vi "ComplexClusterControls.vi"() -> ()   [LabVIEW 2016, in "test_ValueSignal.lvlib"]
uses:
  test_ValueSignal.lvlib
  Helper/HelperVI1.vi
  main/apis/Stimulus/ValueSignalByName.vi
  main/apis/Assert/AssertControlValueByName.vi
  <vilib>/addons/_JKI Toolkits/Caraya/classes/Assert/Assert Equal Value_Variant.vi
  <vilib>/addons/_JKI Toolkits/Caraya/classes/Assert/Assert.lvclass
  <vilib>/addons/_JKI Toolkits/Caraya/classes/Test/Test.lvclass
panel:
  out "error out":errorcluster
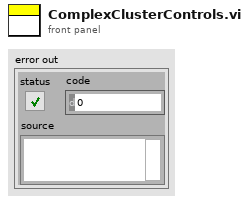
[diagram p1: front panel]
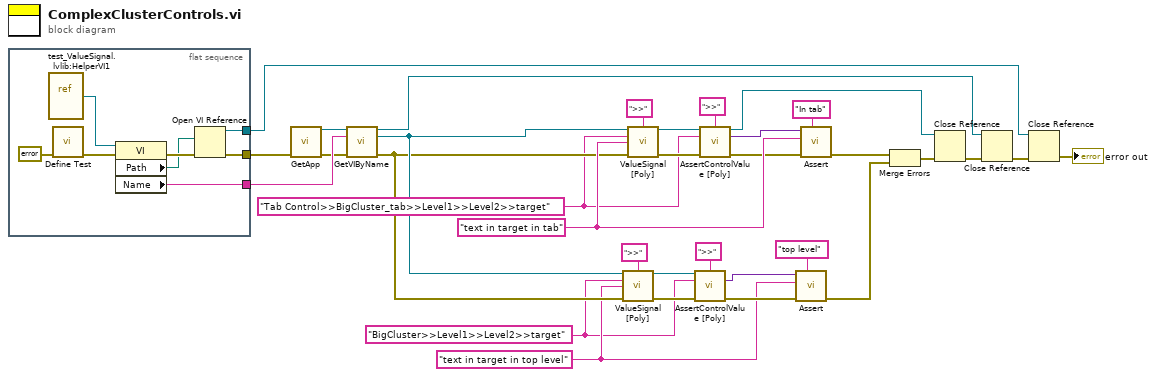
[diagram p0: block diagram]
diagram:
  w3 = "BigCluster>>Level1>>Level2>>target"
  w6 = "Tab Control>>BigCluster_tab>>Level1>>Level2>>target"
  w7 = "text in target in top level"
  w25 = "text in target in tab"
  n1 = flat-sequence {
    tunnel: [w37] -> w28
    tunnel: [w36] -> w30
    tunnel: [w34] -> w27
    frame #0 {
      n2 = vi-ref "test_ValueSignal.lvlib:HelperVI1.vi"() -> (w39:refnum<vi>)
      n3 = call <vilib>:"Define Test.vi"("error in (no error)"=errorcluster {"status"=FALSE, "code"=0, "source"=""}) -> ("error out"=w40:errorcluster)  [unwired: 10 in]
      n4 = property on="Property Node" class="VI"(reference=w39, error in=w40) -> (error out=w38:errorcluster, "Path"=w35:path, "Name"=w34:string)  [unwired: 1 out]
      n5 = Open VI Reference(vi path=w35, error in (no error)=w38) -> (vi reference=w36:refnum<vi>, error out=w37:errorcluster)  [unwired: 4 in]
    }
  }
  n6 = call "GetApp.vi"("error in (no error)"=w28) -> ("Application Ref"=w29:refnum<vi>, "error out"=w26:errorcluster)  [unwired: 13 in]
  n7 = call "GetVIByName.vi"("Application Ref in"=w29, "VI Name"=w27, "error in (no error)"=w26) -> ("Application Ref out"=w9:refnum<vi>, "VI Reference"=w15:refnum<vi>, "error out"=w8:errorcluster)  [unwired: 10 in]
  n8 = call-poly "ValueSignal [Poly].vi"("VI Reference In"=w15, "delimiter (Tab)"=">>", "Control Name"=w3, "Value (Signaling)"=w7, "error in"=w8) -> ("VI Reference Out"=w17:refnum<vi>, "error out"=w18:errorcluster)  [unwired: 9 in]
  n9 = call-poly "ValueSignal [Poly].vi"("VI Reference In"=w15, "delimiter (Tab)"=">>", "Control Name"=w6, "Value (Signaling)"=w25, "error in"=w8) -> ("VI Reference Out"=w24:refnum<vi>, "error out"=w23:errorcluster)  [unwired: 9 in]
  n10 = call-poly "AssertControlValue [Poly].vi"("VI Reference In"=w17, "delimiter (Tab)"=">>", "Control Name"=w3, "error in"=w18) -> ("Value"=w20:variant, "error out"=w19:errorcluster)  [unwired: 9 in, 1 out]
  n11 = call-poly "AssertControlValue [Poly].vi"("VI Reference In"=w24, "delimiter (Tab)"=">>", "Control Name"=w6, "error in"=w23) -> ("VI Reference Out"=w11:refnum<vi>, "Value"=w21:variant, "error out"=w22:errorcluster)  [unwired: 9 in]
  n12 = call-poly <vilib>:"Assert.vi"("Label"="top level" ("Label (VI Title)"), "error in (no error)"=w19, "Y"=w7, "X"=w20) -> ("error out"=w13:errorcluster)  [unwired: 7 in]
  n13 = call-poly <vilib>:"Assert.vi"("Label"="In tab" ("Label (VI Title)"), "error in (no error)"=w22, "Y"=w25, "X"=w21) -> ("error out"=w32:errorcluster)  [unwired: 7 in]
  n14 = Merge Errors(w32, w13) -> (w14:errorcluster)
  n15 = Close Reference(reference=w11, error in (no error)=w14) -> (error out=w12:errorcluster)
  n16 = Close Reference(reference=w9, error in (no error)=w12) -> (error out=w10:errorcluster)
  n17 = Close Reference(reference=w30, error in (no error)=w10) -> (error out=→"error out":errorcluster)
